vi "Average.vi"() -> ()   [LabVIEW 2012]
panel:
  out "Senzori":dbl[](array[numeric])
  out "size(s)":i32
  out "Izlaz iz Bool Niza":u32=16
  in  "Sekvenca":dbl[](array[numeric])
  in  "Treshold":dbl=0.8
  in  "stop":bool
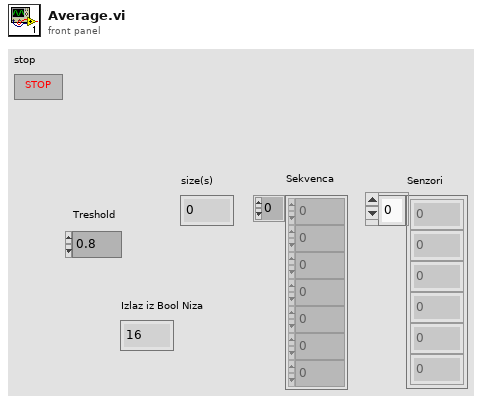
[diagram p1: front panel]
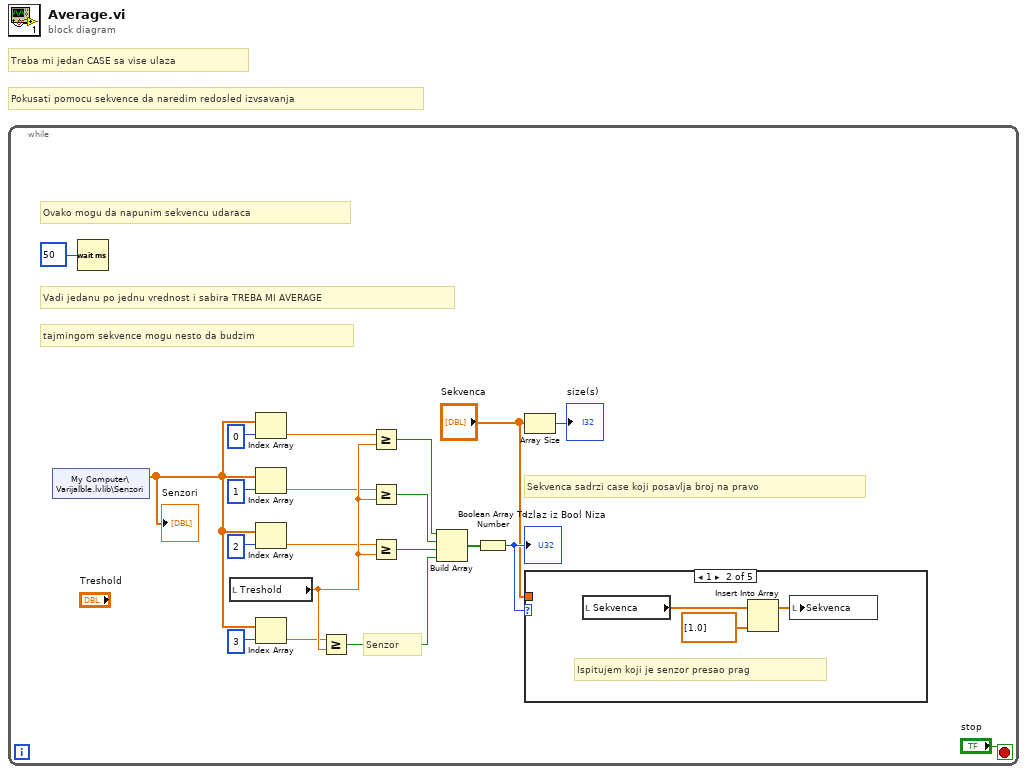
[diagram p0: block diagram]
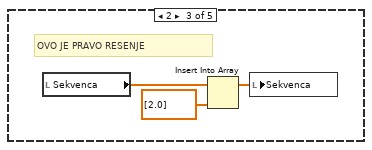
[diagram p3: hidden frame]
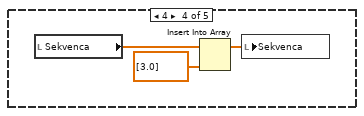
[diagram p4: hidden frame]
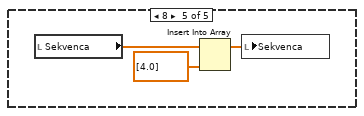
[diagram p5: hidden frame]
diagram:
  # "Pokusati pomocu sekvence da naredim redosled izvsavanja"
  # "Treba mi jedan CASE sa vise ulaza"
  n1 = while {
    stop <- "stop" stop-if-true
    # "Senzor"
    # "Sekvenca sadrzi case koji posavlja broj na pravo"
    # "tajmingom sekvence mogu nesto da budzim"
    # "Ovako mogu da napunim sekvencu udaraca"
    # "Vadi jedanu po jednu vrednost i sabira TREBA MI AVERAGE"
    n2 = shared-variable "My Computer\\Varijalble.lvlib\\Senzori"() -> (w5:dbl[])  [unwired: 1 in, 1 out]
    "Senzori" <- w5
    n3 = Wait (ms)(milliseconds to wait=u32 50) -> ()  [unwired: 1 out]
    n4 = local read "Treshold"() -> (w14:dbl)
    n5 = Index Array(array=w5, index=0) -> (element=w4:dbl)
    n6 = Index Array(array=w5, index=1) -> (element=w3:dbl)
    n7 = Index Array(array=w5, index=2) -> (element=w2:dbl)
    n8 = Index Array(array=w5, index=3) -> (element=w1:dbl)
    n9 = Greater Or Equal?(x=w1, y=w14) -> (x >= y?=w10:bool)
    n10 = Greater Or Equal?(x=w4, y=w14) -> (x >= y?=w13:bool)
    n11 = Greater Or Equal?(x=w3, y=w14) -> (x >= y?=w12:bool)
    n12 = Greater Or Equal?(x=w2, y=w14) -> (x >= y?=w11:bool)
    n13 = Build Array(w13, w12, w11, w10) -> (w9:bool[])
    n14 = Boolean Array To Number(Boolean array=w9) -> (number=w8:u32)
    "Izlaz iz Bool Niza" <- w8
    n15 = Array Size(array="Sekvenca") -> (size(s)=→"size(s)":i32)
    n16 = case shown="1" w8 {
      tunnel: "Sekvenca" -> [_ _ _ _ _]
      frame 0, Default {
      }
      frame 1 {
        # "Ispitujem koji je senzor presao prag"
        n17 = local read "Sekvenca"() -> (w21:dbl[])
        n18 = Insert Into Array(array=w21, new element=dbl[] [1.0]) -> (w23:dbl[])  [unwired: 1 in]
        n19 = local write "Sekvenca"(w23) -> ()
      }
      frame 2 {
        # "OVO JE PRAVO RESENJE"
        n20 = local read "Sekvenca"() -> (w24:dbl[])
        n21 = Insert Into Array(array=w24, new element=dbl[] [2.0]) -> (w26:dbl[])  [unwired: 1 in]
        n22 = local write "Sekvenca"(w26) -> ()
      }
      frame 4 {
        n23 = local read "Sekvenca"() -> (w27:dbl[])
        n24 = Insert Into Array(array=w27, new element=dbl[] [3.0]) -> (w29:dbl[])  [unwired: 1 in]
        n25 = local write "Sekvenca"(w29) -> ()
      }
      frame 8 {
        n26 = local read "Sekvenca"() -> (w30:dbl[])
        n27 = Insert Into Array(array=w30, new element=dbl[] [4.0]) -> (w32:dbl[])  [unwired: 1 in]
        n28 = local write "Sekvenca"(w32) -> ()
      }
    }
  }
